vi "Parametros.vi"(0 "VetorDeDados":dbl[][](array[numeric]), 7 "area":dbl, 9 "irradiancia":dbl, 11 "pontos":dbl) -> (3 "FF":dbl, 4 "Icc":dbl, 6 "Vca":dbl, 8 "Pmp":dbl, 10 "Vmp":dbl, 14 "eficiencia":dbl, 15 "Imp":dbl)   [LabVIEW 2012]
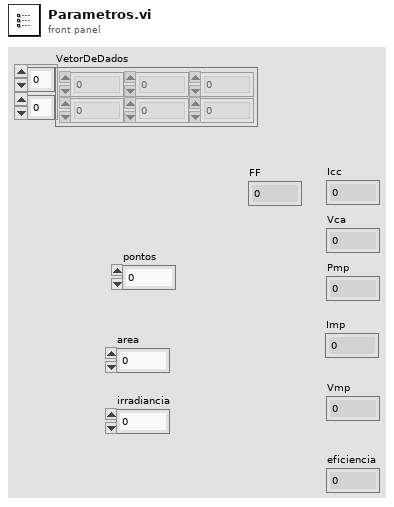
[diagram p1: front panel]
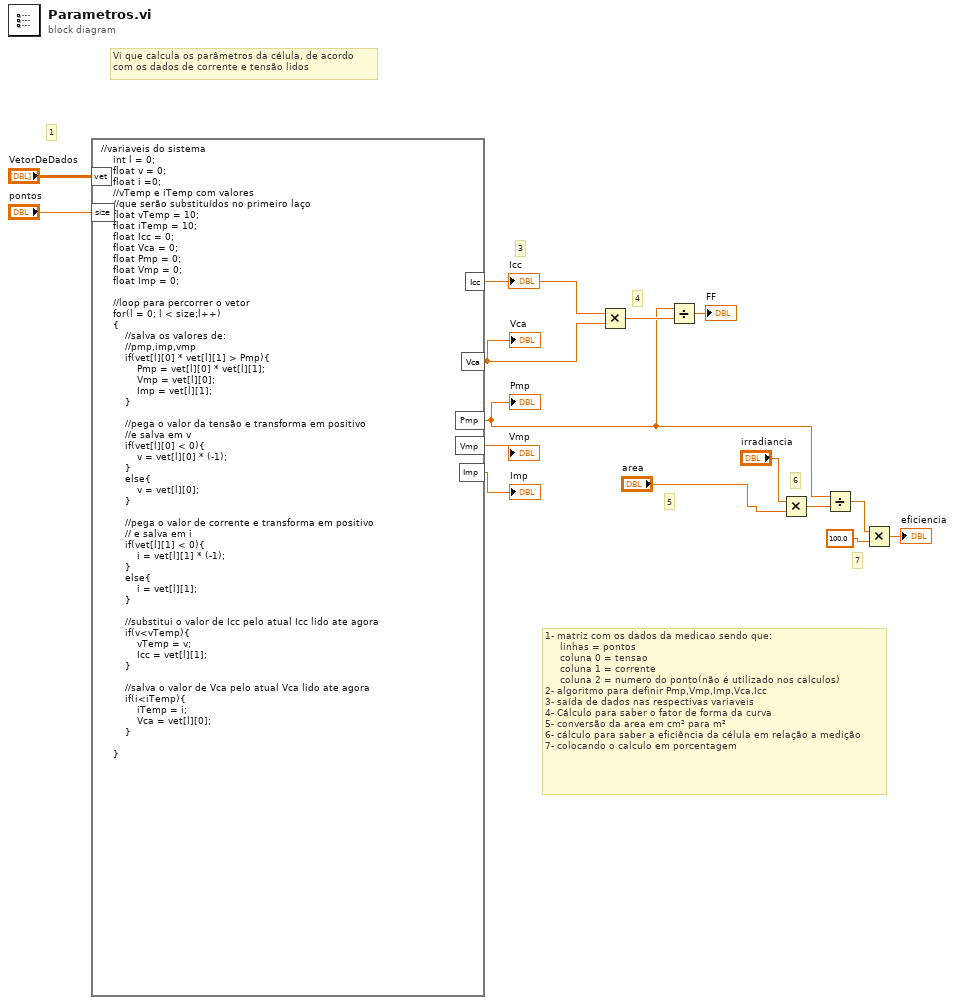
[diagram p0: block diagram]
diagram:
  # "Vi que calcula os parâmetros da célula, de acordo \ncom os dados de corrente e tensão lidos"
  # "5"
  # "1- matriz com os dados da medicao sendo que:\n     linhas = pontos\n     coluna 0 = tensao\n     coluna 1 = corrente\n     coluna 2 = numero do ponto(não é utilizado nos calculos) \n2- algoritmo para definir Pmp,Vmp,Imp,Vca,Icc\n3- saída de dados nas respectivas variaveis\n4- Cálculo para saber o fator de forma da curva\n5- conversão da area em cm² para m²\n6- cálculo para saber a eficiência da célula em relação a medição\n7- colocando o calculo em porcentagem"
  # "6"
  # "4"
  # "3"
  # "2"
  # "1"
  # "7"
  n1 = formula code="//variaveis do sistema\n    int l = 0;\n    float v = 0;\n    float i =0;\n    //vTemp e iTemp com valores\n    //que serão substituídos no primeiro laço\n    float vTemp = 10;\n    float iTemp = 10;\n    float Icc = 0;\n    float Vca = 0;\n    float Pmp = 0;\n    float Vmp = 0;\n    float Imp = 0;\n\n    //loop para percorrer o vetor\n    for(l = 0; l < size;l++)\n    {\n        //salva os valores de:\n        //pmp,imp,vmp\n        if(vet[l][0] * vet[l][1] > Pmp){\n            Pmp = vet[l][0] * vet[l][1];\n            Vmp = vet[l][0];\n            Imp = vet[l][1];\n        }\n\n        //pega o valor da tensão e transforma em positivo\n        //e salva em v\n        if(vet[l][0] < 0){\n            v = vet[l][0] * (-1);\n        }\n        else{\n            v = vet[l][0];\n        }\n\n        //pega o valor de corrente e transforma em positivo\n        // e salva em i\n        if(vet[l][1] < 0){\n            i = vet[l][1] * (-1);\n        }\n        else{\n            i = vet[l][1];\n        }\n        \n        //substitui o valor de Icc pelo atual Icc lido ate agora\n        if(v<vTemp){\n            vTemp = v;\n            Icc = vet[l][1];\n        }\n\n        //salva o valor de Vca pelo atual Vca lido ate agora\n        if(i<iTemp){\n            iTemp = i;\n            Vca = vet[l][0];\n        }\n\n    }"("vet"="VetorDeDados", "size"="pontos") -> ("Icc"=w7:dbl, "Vca"=w6:dbl, "Pmp"=w3:dbl, "Imp"=→"Imp":dbl, "Vmp"=→"Vmp":dbl)
  "Vca" <- w6
  "Pmp" <- w3
  "Icc" <- w7
  n2 = Multiply(x=w7, y=w6) -> (x*y=w5:dbl)
  n3 = Divide(x=w3, y=w5) -> (x/y=→"FF":dbl)
  n4 = Multiply(x="irradiancia", y="area") -> (x*y=w11:dbl)
  n5 = Divide(x=w3, y=w11) -> (x/y=w10:dbl)
  n6 = Multiply(x=w10, y=100.0) -> (x*y=→"eficiencia":dbl)
